vi "M Water Cells.vi"(11 "EV3 in":T1) -> ()   [LabVIEW 2015]
uses:
  <vilib>/NXT/LegoClasses/BrickReference/BrickReference.lvclass
  <vilib>/NXT/Subs/LVHSConnector.ctl
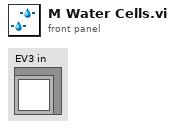
[diagram p1: front panel]
types:
  T1 = typedef "LVHSConnector.ctl" = refnum<class "BrickReference.lvclass">
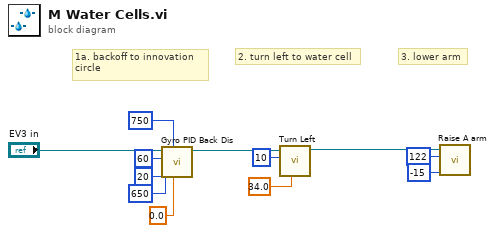
[diagram p0: block diagram]
diagram:
  # "3. lower arm"
  # "2. turn left to water cell"
  # "1a. backoff to innovation\ncircle"
  n1 = call "Gyro PID Back Dis.vi"("Target angle"=sgl 0.0, "Threshold to stop"=750, "Threshold to slow"=650, "Min. speed"=20, "Max. speed"=60, "EV3 in"="EV3 in") -> ("EV3 out"=w7:T1)  [unwired: 5 in]
  n2 = call "Turn Left.vi"("Turning angle"=sgl 34.0, "Motor B (right)"=i8 10, "EV3 in"=w7) -> ("EV3 out"=w4:T1)  [unwired: 8 in]
  n3 = call "Raise A arm.vi"("Power"=i8 -15, "Rotation"=122, "EV3 in"=w4) -> ()  [unwired: 8 in, 1 out]
